vi "UDP Read and adjust input size.vi"(8 "error in (no error)":errorcluster, 9 "Estimated input size":i32, 10 "Input Size Delta":i32, 11 "connection ID":refnum<k16>) -> (0 "error out":errorcluster, 1 "Estimated input size out":i32, 2 "data out":string, 3 "connection ID out":refnum<k16>)   [LabVIEW 2015, in "E2E Runtime (UDP).lvclass"]
uses:
  E2E Runtime (UDP).lvclass
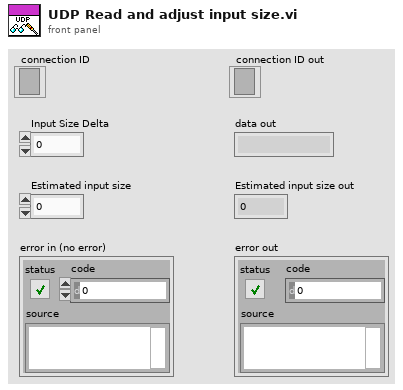
[diagram p1: front panel]
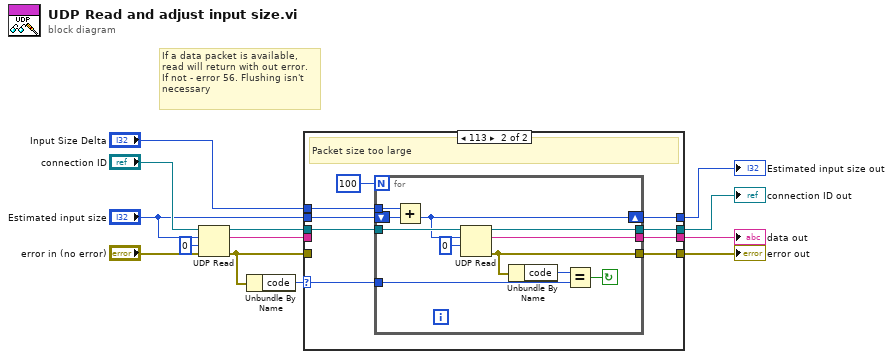
[diagram p0: block diagram]
diagram:
  # "If a data packet is available,\nread will return with out error.\nIf not - error 56. Flushing isn't\nnecessary"
  n1 = UDP Read(connection ID="connection ID", max size (548)="Estimated input size", timeout ms (25000)=0, 8:"error in (no error)") -> (data out=w13:string, error out=w11:errorcluster, 3:w10:refnum<k16>)  [unwired: 2 out]
  n2 = Unbundle By Name(w11) -> ("code"=w12:i32)
  n3 = case shown="113" w12 {
    selector: w12 -> [_ w24]
    tunnel: w11 -> [w17 _]
    tunnel: [w17 w22] -> w9
    tunnel: w10 -> [w15 w26]
    tunnel: w13 -> [w16 _]
    tunnel: [w16 w23] -> w4
    tunnel: [w15 w21] -> w5
    tunnel: "Input Size Delta" -> [_ w20]
    tunnel: "Estimated input size" -> [w14 w19]
    tunnel: [w14 w18] -> w1
    frame Default {
    }
    frame 113 {
      # "Packet size too large"
      n4 = for {
        N: 100 -> [_]
        tunnel: [w36] -> w22
        tunnel: w24 -> [w33]
        tunnel: [w31] -> w23
        tunnel: w26 -> [w37]
        tunnel: [w30] -> w21
        tunnel: w20 -> [w29]
        shift-right: [w27] -> w18
        shift-left: w19 -> [w28]
        stop <- w32 continue-if-true
        n5 = Add(x=w29, y=w28) -> (x+y=w27:i32)
        n6 = UDP Read(connection ID=w37, max size (548)=w27, timeout ms (25000)=0) -> (data out=w31:string, error out=w36:errorcluster, 3:w30:refnum<k16>)  [unwired: 1 in, 2 out]
        n7 = Unbundle By Name(w36) -> ("code"=w34:i32)
        n8 = Equal?(x=w34, y=w33) -> (x = y?=w32:bool)
      }
    }
  }
  "error out" <- w9
  "connection ID out" <- w5
  "data out" <- w4
  "Estimated input size out" <- w1
